vi "Command Timing.vi"(8 "error in (no error)":errorcluster, 9 "Seconds":dbl format="%.6f", 10 "Command":string) -> (0 "error out":errorcluster, 2 "Status Time":dbl format="%.4f", 3 "Comand Timing out":cluster{"Command":string, "Seconds":dbl}[](array[cluster]) {"Seconds" format="%.6f"})   [LabVIEW 2020]
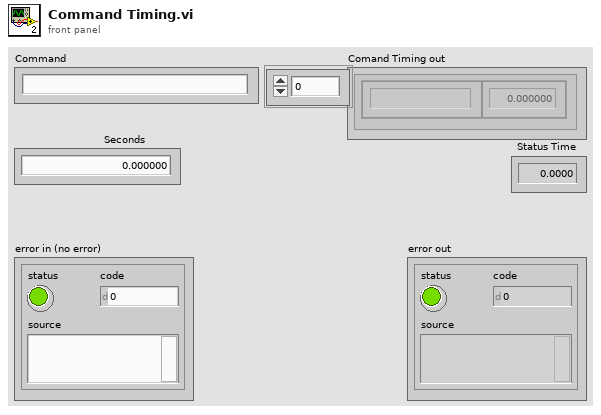
[diagram p1: front panel]
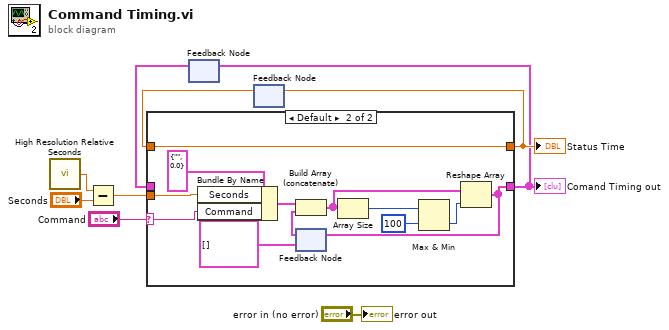
[diagram p0: block diagram]
diagram:
  n1 = call <vilib>:"High Resolution Relative Seconds.vi"() -> ("relative seconds"=w8:dbl)
  n2 = Subtract(x=w8, y="Seconds") -> (x-y=w7:dbl)
  n3 = feedback #1() -> (w3:cluster{"Command":string, "Seconds":dbl}[])  [unwired: 1 in]
  n4 = feedback #2() -> (w4:dbl)  [unwired: 1 in]
  n5 = case shown="Default" "Command" {
    selector: "Command" -> [_ w14]
    tunnel: w7 -> [w11 w18]
    tunnel: [w10 w16] -> w1
    tunnel: [w11 w15] -> w2
    tunnel: w4 -> [_ w15]
    tunnel: w3 -> [w10 _]
    frame "Status" {
    }
    frame Default {
      n6 = Bundle By Name(cluster=cluster{"Command":string, "Seconds":dbl} {"Command"="", "Seconds"=0.0} ("Timing"), "Seconds"=w18, "Command"=w14) -> (w23:cluster{"Command":string, "Seconds":dbl})
      n7 = feedback #3(cluster{"Command":string, "Seconds":dbl}[] [] ("Comand Timing out")) -> (w17:cluster{"Command":string, "Seconds":dbl}[])
      n8 = Build Array (concatenate)(w23, w17) -> (w20:cluster{"Command":string, "Seconds":dbl}[])
      n9 = Array Size(array=w20) -> (size(s)=w22:i32)
      n10 = Max & Min(x=w22, y=100) -> (min(x,y)=w19:i32)  [unwired: 1 out]
      n11 = Reshape Array(w20, w19) -> (w16:cluster{"Command":string, "Seconds":dbl}[])
      n12 = feedback-in #3(w16) -> ()
    }
  }
  "Comand Timing out" <- w1
  "Status Time" <- w2
  n13 = feedback-in #1(w1) -> ()
  n14 = feedback-in #2(w2) -> ()
  "error out" <- "error in (no error)"
